vi "multimeter.vi"() -> ()   [LabVIEW 2024]
uses:
  <vilib>/Utility/file.llb/Write Delimited Spreadsheet (DBL).vi
  <vilib>/ptbypt/NI_PtbyPt.lvlib
  <vilib>/Analysis/NI_AALPro.lvlib
panel:
  out "cluster":cluster{"Numeric":dbl, "mean":dbl}
  out "return count":u32
  out "XY Graph":cluster{"time":dbl[], "values":dbl[]}(graph)
  out "Waveform Chart":cluster{"Numeric":dbl, "mean":dbl}(graph)
  in  "# bins":i32
  in  "min":dbl format="%0.2f"
  in  "max":dbl format="%0.2f"
  out "Histogram":T1(graph)
  out "Numeric":dbl
  out "read buffer":string
  in  "Light intensity [%]":dbl(ramp)
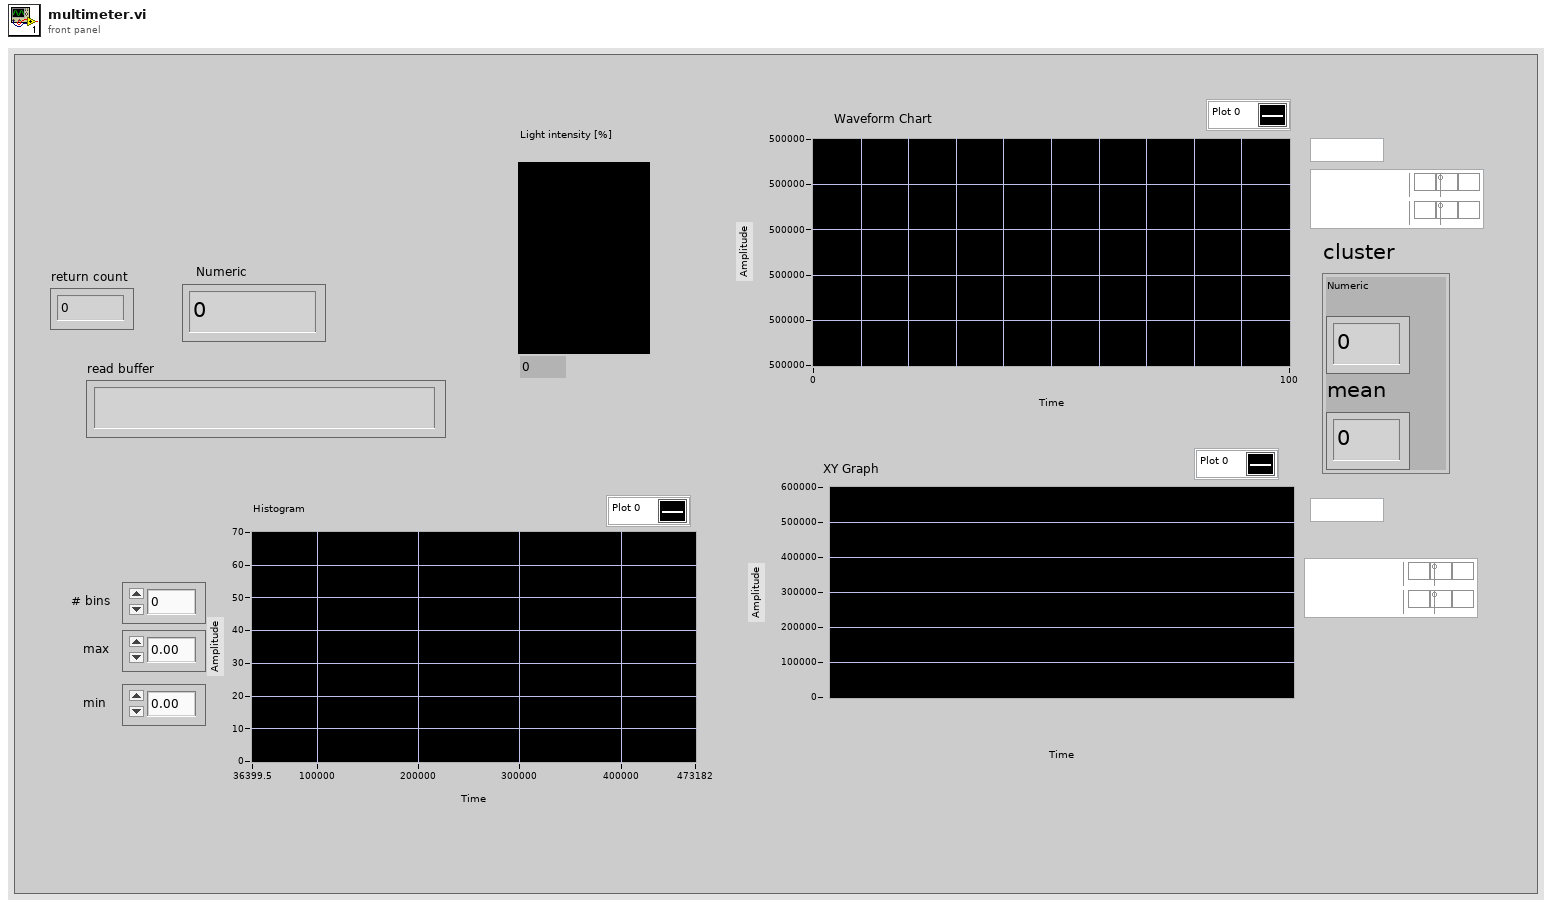
[diagram p1: front panel]
types:
  T1 = cluster{"X Values":dbl[], "Histogram: h(x)":i32[]}
  T2 = enum16{"Configure Port", "Write", "Read", "Close"}
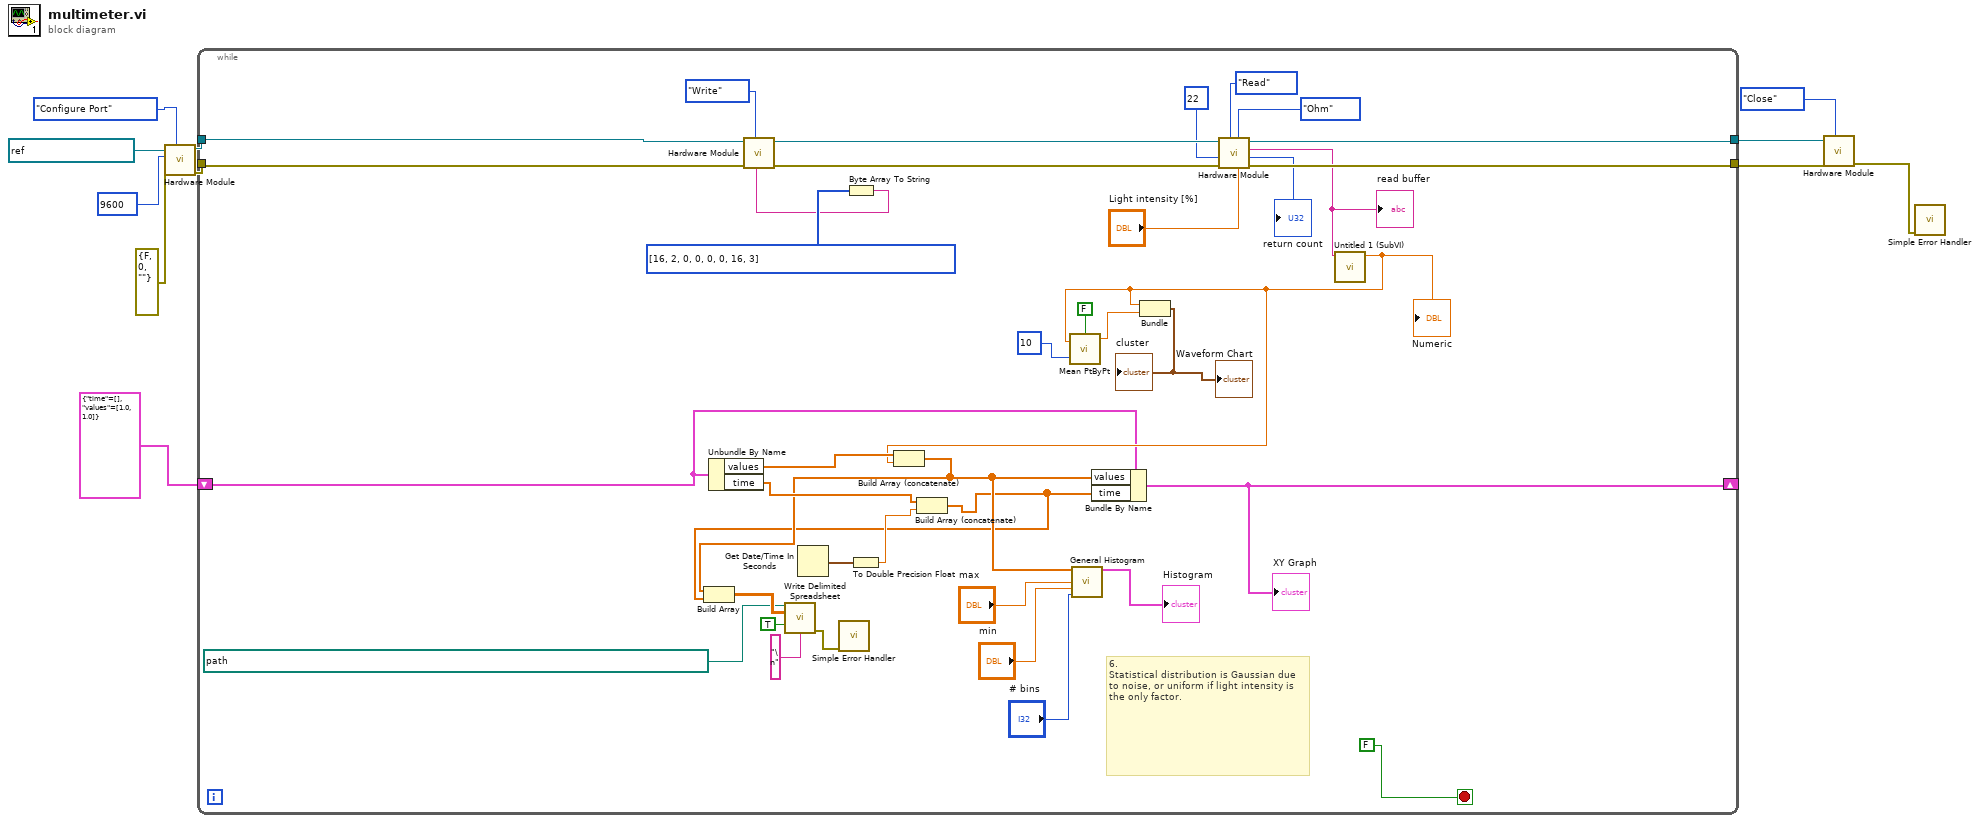
[diagram p0: block diagram]
diagram:
  n1 = call "Hardware Module.vi"("State"=T2."Configure Port", "error in (no error)"=errorcluster {"status"=FALSE, "code"=0, "source"=""}, "baud rate (9600)"=u32 9600, "VISA resource name"=refnum<visa-resource-name> "VirtualDevice1") -> ("error out"=w8:errorcluster, "VISA resource name out"=w7:refnum<visa-resource-name>)  [unwired: 4 in, 2 out]
  n2 = while {
    tunnel: w8 -> [w40]
    tunnel: w7 -> [w39]
    tunnel: [w38] -> w4
    tunnel: [w37] -> w3
    shift-right: [w21] -> _
    shift-left: cluster{"time":dbl[], "values":dbl[]} {"time"=[], "values"=[1.0, 1.0]} ("input cluster") -> [w25]
    stop <- FALSE stop-if-true
    # "6.\nStatistical distribution is Gaussian due to noise, or uniform if light intensity is the only factor."
    n3 = Unbundle By Name(w25) -> ("values"=w32:dbl[], "time"=w31:dbl[])
    n4 = Get Date/Time In Seconds() -> (seconds since 1Jan1904=w41:timestamp)
    n5 = Byte Array To String(unsigned byte array=i32[] [16, 2, 0, 0, 0, 0, 16, 3]) -> (string=w42:string)
    n6 = call "Hardware Module.vi"("write buffer"=w42, "State"=T2."Write", "error in (no error)"=w40, "VISA resource name"=w39) -> ("error out"=w48:errorcluster, "VISA resource name out"=w49:refnum<visa-resource-name>)  [unwired: 4 in, 2 out]
    n7 = To Double Precision Float(number=w41) -> (double precision float=w30:dbl)
    n8 = Build Array (concatenate)(w31, w30) -> (w18:dbl[])
    n9 = call "Hardware Module.vi"("Light intensity [%]"="Light intensity [%]", "Mode"=enum16{"Ohm", "DcV"}."Ohm", "State"=T2."Read", "error in (no error)"=w48, "byte count"=u32 22, "VISA resource name"=w49) -> ("error out"=w38:errorcluster, "return count"=→"return count":u32, "read buffer"=w26:string, "VISA resource name out"=w37:refnum<visa-resource-name>)  [unwired: 2 in]
    "read buffer" <- w26
    n10 = call "Untitled 1 (SubVI).vi"("read buffer"=w26) -> ("Numeric"=w27:dbl)  [unwired: 10 in]
    "Numeric" <- w27
    n11 = Build Array (concatenate)(w32, w27) -> (w19:dbl[])
    n12 = Build Array(w19, w18) -> (w17:dbl[][])
    n13 = call-poly <vilib>:"Write Delimited Spreadsheet.vi"("file path (dialog if empty)"=path "C:/Users/left4/OneDrive/Masaüstü/comp measur labs/multimeter/Data.txt", "2D data"=w17, "append to file? (new file:F)"=TRUE, "delimiter (\\t)"="\n" ("delimiter (\\t)")) -> ("error out"=w20:errorcluster)  [unwired: 10 in, 1 out]
    n14 = call <vilib>:"Simple Error Handler.vi"("error in (no error)"=w20) -> ()  [unwired: 4 in, 5 out]
    n15 = call <vilib>:"Mean PtByPt.vi"("x"=w27, "sample length"=10, "initialize"=FALSE) -> ("mean"=w24:dbl)  [unwired: 1 in, 1 out]
    n16 = call <vilib>:"General Histogram.vi"("X"=w19, "max"="max", "min"="min", "# bins"="# bins") -> ("Histogram Graph"=→"Histogram":T1)  [unwired: 7 in, 4 out]
    n17 = Bundle By Name(cluster=w25, "values"=w19, "time"=w18) -> (w21:cluster{"time":dbl[], "values":dbl[]})
    "XY Graph" <- w21
    n18 = Bundle("Numeric"=w27, "mean"=w24) -> (→"Waveform Chart" →"cluster":cluster{"Numeric":dbl, "mean":dbl})  [unwired: 1 in]
  }
  n19 = call "Hardware Module.vi"("State"=T2."Close", "error in (no error)"=w4, "VISA resource name"=w3) -> ("error out"=w1:errorcluster)  [unwired: 5 in, 3 out]
  n20 = call <vilib>:"Simple Error Handler.vi"("error in (no error)"=w1) -> ()  [unwired: 4 in, 5 out]
